vi "Test.vi"() -> ()   [LabVIEW 2018, in "Potentiostat Galvanostat.lvclass"]
uses:
  Potentiostat Galvanostat.lvclass
  Controls/OCV Parameters.ctl
  Controls/CV Parameters.ctl
  Controls/CA Parameters.ctl
  Controls/CP Parameters.ctl
  Controls/PEIS Parameters.ctl
  Controls/GEIS Parameters.ctl
  Controls/Channel Information.ctl
  Controls/Channel.ctl
  Controls/Firmware Code.ctl
  Controls/Amplifier Type.ctl
  Controls/Channel State.ctl
  Controls/Current Range.ctl
  Controls/Bandwidth.ctl
  Controls/Device Information.ctl
  Controls/Device Code.ctl
  Controls/Technique List.ctl
  Controls/PEIS-GEIS P1 Processed Data Columns.ctl
  Potentiostat Galvanostat.lvclass/Potentiostat Galvanostat.ctl
  Error Code Converter.vi
  Insert Column into Table.vi
  BL_GetErrorMsg.vi
  <vilib>/Utility/error.llb/Error Cluster From Error Code.vi
  Get Enum Size.vi
  <vilib>/Utility/Data Type/Get Numeric Information.vi
panel:
  out "Version":string="6.4.0.0"
  out "Device Information":T1={"Device Code"=36, "RAM Size"=32, "CPU"=9200, "Number Of Channels"=2, "Number Of Slots"=1, "Firmware Version"=1140, "Firmware Year"=2021, "Firmware Month"=6, "Firmware Day"=17, "HT Display On"=1, "No. of Connected PCs"=1} {"Device Code" items=["VMP device"=0, "VMP2 device"=1, "MPG device"=2, "BISTAT device"=3, "MCS-200 device"=4, "VMP3 device"=5, "VSP"=6, "HCP-803"=7, "EPP-400"=8, "EPP-4000"=9, "BISTAT 2"=10, "FCT-150S"=11, "VMP-300"=12, "SP-50"=13, "SP-150"=14, "FCT-50S"=15, "SP300"=16, "CLB-500"=17, "HCP-1005"=18, "CLB-2000"=19, "VSP-300"=20, "SP-200"=21, "MPG2"=22, "SP-100"=23, "MOSLED"=24, "Kinetic device... \\warning unused code"=25, "Nikita"=26, "SP-240"=27, "MPG-205 (techno VMP3) \\warning not controled by kernel2"=28, "MPG-210 (techno VMP3) \\warning not controled by kernel2"=29, "MPG-220 (techno VMP3) \\warning not controled by kernel2"=30, "MPG-240 (techno VMP3) \\warning not controled by kernel2"=31, "BP-300"=32, "VMP-3e  (VMP3)"=33, "VSP-3e  (VMP3)"=34, "SP-50e  (VMP3)"=35, "SP-150e (VMP3)"=36, "Unknown device"=255]}
  out "Channel Information":T3={"Channel"=0, "Board Version"=19, "Board Serial Number"=54353, "Firmware Code"=5, "Firmware Version"=5282, "Xilinx Version"=42511, "Amplifier Code"=15, "Number of Amplifiers"=0, "Low Current Board Present?"=FALSE, "Impedance Capable?"=TRUE, "RESERVED"=0, "RESERVED 2"=0, "Memory Size"=786432, "Memory Filled (in Bytes)"=0, "Channel State"=0, "Maximum Current Range Allowed"=10, "Minimum Current Range Allowed"=5, "Maximum Bandwidth"=7, "Number of Techniques"=1} {"Channel" items=["Channel 0", "Channel 1", "Channel 2", "Channel 3", "Channel 4", "Channel 5", "Channel 6", "Channel 7", "Channel 8", "Channel 9", "Channel 10", "Channel 11", "Channel 12", "Channel 13", "Channel 14", "Channel 15"]; "Firmware Code" items=["No firmware loaded"=0, "Firmware for EC-Lab software"=1, "Unknown firmware loaded"=4, "Firmware for the library"=5, "Invalid firmware loaded"=8, "Firmware for calibration software"=10]; "Amplifier Code" items=["No amplifier VMP3 series"=0, "Amplifier 2 A VMP3 series"=1, "Amplifier 1 A VMP3 series"=2, "Amplifier 5 A VMP3 series"=3, "Amplifier 10 A VMP3 series"=4, "Amplifier 20 A VMP3 series"=5, "reserved VMP3 series"=6, "Low current amplifier VMP3 series"=7, "Amplifier 80 A VMP3 series"=8, "Amplifier 4 A VMP3 series"=9, "Fuel Cell Tester VMP3 series"=10, "Amplifier 4 A (VSP instrument) VMP3 series"=11, "Low current amplifier (VSP instrument) VMP3 series"=12, "Undefined amplifier VMP3 series"=13, "reserved VMP3 series"=14, "No amplifier VMP3 series"=15, "Amplifier 8 A VMP3 series"=16, "Amplifier LB500 VMP3 series"=17, "Amplifier 100 A VMP3 series"=18, "Amplifier LB2000 VMP3 series"=19, "Amplifier 1A 48V SP-300 series"=20, "Amplifier 4A 14V SP-300 series"=21, "MPG-205 5A amplifier"=22, "MPG-210 10A amplifier"=23, "MPG-220 20A amplifier"=24, "MPG-240 40A amplifier"=25, "coin cell holder"=26, "VMP4 10A/5V amplifier (SP-300 internal amplifier)"=27, "VMP4 2A/30V"=28, "VMP4 1A/48VP"=129]; "Channel State" items=["Channel is stopped", "Channel is running", "Channel is paused"]; "Maximum Current Range Allowed" items=["I range 100 pA SP-300 series", "I range 1 nA VMP3 / SP-300 series", "I range 10 nA VMP3 / SP-300 series", "I range 100 nA VMP3 / SP-300 series", "I range 1 uA VMP3 / SP-300 series", "I range 10 uA VMP3 / SP-300 series", "I range 100 uA VMP3 / SP-300 series", "I range 1 mA VMP3 / SP-300 series", "I range 10 mA VMP3 / SP-300 series", "I range 100 mA VMP3 / SP-300 series", "I range 1 A VMP3 / SP-300 series", "Booster VMP3 / SP-300 series", "Auto range VMP3 / SP-300 series"]; "Minimum Current Range Allowed" items=["I range 100 pA SP-300 series", "I range 1 nA VMP3 / SP-300 series", "I range 10 nA VMP3 / SP-300 series", "I range 100 nA VMP3 / SP-300 series", "I range 1 uA VMP3 / SP-300 series", "I range 10 uA VMP3 / SP-300 series", "I range 100 uA VMP3 / SP-300 series", "I range 1 mA VMP3 / SP-300 series", "I range 10 mA VMP3 / SP-300 series", "I range 100 mA VMP3 / SP-300 series", "I range 1 A VMP3 / SP-300 series", "Booster VMP3 / SP-300 series", "Auto range VMP3 / SP-300 series"]; "Maximum Bandwidth" items=["Bandwidth #1"=1, "Bandwidth #2"=2, "Bandwidth #3"=3, "Bandwidth #4"=4, "Bandwidth #5"=5, "Bandwidth #6"=6, "Bandwidth #7"=7, "Bandwidth #8 (only with SP-300 series)"=8, "Bandwidth #9 (only with SP-300 series)"=9]}
  out "Plugged Channels":u8[](array[ring])=[0, 1] items=["Channel 0", "Channel 1", "Channel 2", "Channel 3", "Channel 4", "Channel 5", "Channel 6", "Channel 7", "Channel 8", "Channel 9", "Channel 10", "Channel 11", "Channel 12", "Channel 13", "Channel 14", "Channel 15"]
  in  "Stop":bool
  out "Process 1 Table":string[][](table)=[["1.000156E+5", "8.985447E-3", "1.609175E-5", "-3.228165E-1", "-8.278794E-4", "2.261308E-7", "0.000000E+0", "1.676092E-2", "1.613657E-5", "-1.723862E-1", "8.918704E-4", "-2.261308E-7", "0.000000E+0", "1.913000E+0", "1.000001E+0", "5.000068E+0", "-4.793397E+0", "-4.792189E+0", "-1.849602E+1", "-9.877000E+0", "5.583884E+2", "1.038692E+3", "2.746936E+0", "3.016487E+0", "1.771425E+2", "1.781706E+2", "5.295453E+2", "1.023296E+3"], ["7.942968E+4", "9.130012E-3", "1.555612E-5", "-3.760847E-1", "-8.272454E-4", "2.359809E-7", "0.000000E+0", "1.656449E-2", "1.558345E-5", "-2.054282E-1", "8.834808E-4", "-2.359809E-7", "0.000000E+0", "2.200000E+0", "1.000001E+0", "4.899983E+0", "-4.808099E+0", "-4.807336E+0", "-2.154807E+1", "-1.177017E+1", "5.869082E+2", "1.062954E+3", "2.768570E+0", "3.026514E+0", "2.155606E+2", "2.168281E+2", "5.458891E+2", "1.040604E+3"], ["6.309374E+4", "9.176587E-3", "1.457716E-5", "-4.301943E-1", "-8.320003E-4", "2.343205E-7", "0.000000E+0", "1.605249E-2", "1.459336E-5", "-2.420709E-1", "8.697778E-4", "-2.343205E-7", "0.000000E+0", "2.487000E+0", "1.000001E+0", "4.799986E+0", "-4.836327E+0", "-4.835845E+0", "-2.464832E+1", "-1.386964E+1", "6.295180E+2", "1.099986E+3", "2.799008E+0", "3.041387E+0", "2.625389E+2", "2.636817E+2", "5.721593E+2", "1.067915E+3"], ["5.011718E+4", "9.267574E-3", "1.345851E-5", "-4.798813E-1", "-8.280845E-4", "2.151425E-7", "0.000000E+0", "1.554337E-2", "1.346797E-5", "-2.804208E-1", "8.782047E-4", "-2.151425E-7", "0.000000E+0", "2.774000E+0", "1.000001E+0", "4.699987E+0", "-4.871003E+0", "-4.870698E+0", "-2.749517E+1", "-1.606693E+1", "6.886035E+2", "1.154099E+3", "2.837969E+0", "3.062243E+0", "3.179103E+2", "3.194085E+2", "6.108256E+2", "1.109019E+3"], ["3.981250E+4", "9.361682E-3", "1.227965E-5", "-5.128311E-1", "-8.262572E-4", "2.463346E-7", "0.000000E+0", "1.500565E-2", "1.228510E-5", "-3.115016E-1", "8.827538E-4", "-2.463346E-7", "0.000000E+0", "3.061000E+0", "1.000001E+0", "4.600019E+0", "-4.910814E+0", "-4.910621E+0", "-2.938306E+1", "-1.784773E+1", "7.623738E+2", "1.221452E+3", "2.882168E+0", "3.086876E+0", "3.740558E+2", "3.743606E+2", "6.643013E+2", "1.162668E+3"], ["3.162500E+4", "9.495218E-3", "1.114971E-5", "-5.244131E-1", "-8.288304E-4", "2.266156E-7", "0.000000E+0", "1.457268E-2", "1.115284E-5", "-3.323534E-1", "8.945179E-4", "-2.266156E-7", "0.000000E+0", "3.348000E+0", "1.000001E+0", "4.500030E+0", "-4.952736E+0", "-4.952614E+0", "-3.004666E+1", "-1.904244E+1", "8.516111E+2", "1.306634E+3", "2.930241E+0", "3.116154E+0", "4.264060E+2", "4.263136E+2", "7.371698E+2", "1.235131E+3"], ["2.511718E+4", "9.653487E-3", "1.011711E-5", "-5.154602E-1", "-8.220057E-4", "2.375851E-7", "0.000000E+0", "1.425756E-2", "1.011891E-5", "-3.393087E-1", "8.821572E-4", "-2.375851E-7", "0.000000E+0", "3.635000E+0", "1.000001E+0", "4.399971E+0", "-4.994943E+0", "-4.994866E+0", "-2.953369E+1", "-1.944096E+1", "9.541741E+2", "1.409001E+3", "2.979628E+0", "3.148911E+0", "4.703461E+2", "4.689655E+2", "8.301944E+2", "1.328667E+3"], ["1.995312E+4", "9.780001E-3", "9.222543E-6", "-4.890218E-1", "-8.317952E-4", "2.165788E-7", "0.000000E+0", "1.401417E-2", "9.223570E-6", "-3.334392E-1", "8.876571E-4", "-2.165788E-7", "0.000000E+0", "3.922000E+0", "1.000001E+0", "4.300011E+0", "-5.035149E+0", "-5.035101E+0", "-2.801888E+1", "-1.910466E+1", "1.060445E+3", "1.519386E+3", "3.025488E+0", "3.181668E+0", "4.981574E+2", "4.972872E+2", "9.361534E+2", "1.435702E+3"], ["1.585156E+4", "8.546229E-3", "7.339862E-6", "-4.445049E-1", "-8.202157E-4", "2.327903E-7", "0.000000E+0", "1.195757E-2", "7.340385E-6", "-3.115652E-1", "8.815979E-4", "-2.327904E-7", "0.000000E+0", "4.066000E+0", "1.000001E+0", "4.200072E+0", "-5.134312E+0", "-5.134281E+0", "-2.546825E+1", "-1.785137E+1", "1.164358E+3", "1.629012E+3", "3.066087E+0", "3.211924E+0", "5.006867E+2", "4.993717E+2", "1.051210E+3", "1.550583E+3"], ["1.258594E+4", "9.176141E-3", "7.330036E-6", "-3.901606E-1", "-8.220244E-4", "2.196195E-7", "0.000000E+0", "1.263255E-2", "7.330360E-6", "-2.791597E-1", "8.822691E-4", "-2.196195E-7", "0.000000E+0", "4.210000E+0", "1.000001E+0", "4.099886E+0", "-5.134894E+0", "-5.134875E+0", "-2.235455E+1", "-1.599467E+1", "1.251855E+3", "1.723320E+3", "3.097554E+0", "3.236366E+0", "4.761266E+2", "4.748572E+2", "1.157775E+3", "1.656605E+3"], ["1.001563E+4", "9.575242E-3", "7.255554E-6", "-3.389324E-1", "-8.267233E-4", "2.229029E-7", "0.000000E+0", "1.302152E-2", "7.255760E-6", "-2.448211E-1", "8.815420E-4", "-2.229029E-7", "0.000000E+0", "4.354000E+0", "1.000001E+0", "4.000678E+0", "-5.139329E+0", "-5.139317E+0", "-1.941940E+1", "-1.402721E+1", "1.319712E+3", "1.794646E+3", "3.120479E+0", "3.253979E+0", "4.387784E+2", "4.349913E+2", "1.244634E+3", "1.741131E+3"], ["7.944258E+3", "9.838177E-3", "7.131193E-6", "-2.801160E-1", "-8.239449E-4", "2.293017E-7", "0.000000E+0", "1.327432E-2", "7.131322E-6", "-2.053436E-1", "8.777387E-4", "-2.293017E-7", "0.000000E+0", "4.499000E+0", "1.000001E+0", "3.900053E+0", "-5.146838E+0", "-5.146830E+0", "-1.604946E+1", "-1.176532E+1", "1.379598E+3", "1.861411E+3", "3.139752E+0", "3.269842E+0", "3.814133E+2", "3.795483E+2", "1.325826E+3", "1.822305E+3"], ["6.310570E+3", "9.992450E-3", "7.024918E-6", "-2.357731E-1", "-8.496587E-4", "1.880729E-7", "0.000000E+0", "1.339510E-2", "7.024993E-6", "-1.738710E-1", "8.380091E-4", "-1.880729E-7", "0.000000E+0", "4.676000E+0", "1.000001E+0", "3.800069E+0", "-5.153359E+0", "-5.153354E+0", "-1.350880E+1", "-9.962077E+0", "1.422429E+3", "1.906778E+3", "3.153031E+0", "3.280300E+0", "3.322720E+2", "3.298655E+2", "1.383076E+3", "1.878028E+3"], ["5.013020E+3", "1.008475E-2", "6.978094E-6", "-1.941717E-1", "-8.439901E-4", "1.961507E-7", "0.000000E+0", "1.349288E-2", "6.978146E-6", "-1.427641E-1", "8.002557E-4", "-1.961508E-7", "0.000000E+0", "4.891000E+0", "1.000001E+0", "3.700099E+0", "-5.156263E+0", "-5.156260E+0", "-1.112522E+1", "-8.179780E+0", "1.445201E+3", "1.933591E+3", "3.159928E+0", "3.286365E+0", "2.788571E+2", "2.751105E+2", "1.418043E+3", "1.913919E+3"], ["3.981370E+3", "1.014667E-2", "6.926322E-6", "-1.626481E-1", "-8.424984E-4", "1.827560E-7", "0.000000E+0", "1.355241E-2", "6.926357E-6", "-1.222966E-1", "8.025489E-4", "-1.827560E-7", "0.000000E+0", "5.105000E+0", "1.000001E+0", "3.600032E+0", "-5.159497E+0", "-5.159495E+0", "-9.319052E+0", "-7.007077E+0", "1.464943E+3", "1.956644E+3", "3.165821E+0", "3.291512E+0", "2.372212E+2", "2.386948E+2", "1.445609E+3", "1.942030E+3"], ["3.160056E+3", "1.018775E-2", "6.921268E-6", "-1.311982E-1", "-8.471414E-4", "1.910018E-7", "0.000000E+0", "1.357444E-2", "6.921282E-6", "-9.735066E-2", "8.062589E-4", "-1.910018E-7", "0.000000E+0", "5.319000E+0", "1.000001E+0", "3.499695E+0", "-5.159814E+0", "-5.159813E+0", "-7.517101E+0", "-5.577782E+0", "1.471948E+3", "1.961262E+3", "3.167893E+0", "3.292536E+0", "1.925634E+2", "1.906287E+2", "1.459298E+3", "1.951976E+3"], ["2.514022E+3", "1.021940E-2", "6.880800E-6", "-1.155739E-1", "-8.465820E-4", "1.765624E-7", "0.000000E+0", "1.358598E-2", "6.880814E-6", "-8.642459E-2", "8.008709E-4", "-1.765624E-7", "0.000000E+0", "5.533000E+0", "1.000001E+0", "3.400369E+0", "-5.162361E+0", "-5.162360E+0", "-6.621896E+0", "-4.951764E+0", "1.485206E+3", "1.974472E+3", "3.171787E+0", "3.295451E+0", "1.712691E+2", "1.704306E+2", "1.475298E+3", "1.967103E+3"], ["1.993189E+3", "1.022407E-2", "6.874916E-6", "-1.008002E-1", "-8.456683E-4", "1.845843E-7", "0.000000E+0", "1.360339E-2", "6.874928E-6", "-7.507443E-2", "8.015048E-4", "-1.845843E-7", "0.000000E+0", "5.748000E+0", "1.000001E+0", "3.299548E+0", "-5.162733E+0", "-5.162732E+0", "-5.775424E+0", "-4.301448E+0", "1.487155E+3", "1.978695E+3", "3.172356E+0", "3.296379E+0", "1.496518E+2", "1.484099E+2", "1.479606E+3", "1.973121E+3"], ["1.582532E+3", "1.023726E-2", "6.832585E-6", "-8.925927E-2", "-8.457801E-4", "1.719544E-7", "0.000000E+0", "1.360714E-2", "6.832587E-6", "-6.638539E-2", "8.021015E-4", "-1.719544E-7", "0.000000E+0", "5.963000E+0", "1.000001E+0", "3.199352E+0", "-5.165415E+0", "-5.165415E+0", "-5.114179E+0", "-3.803603E+0", "1.498300E+3", "1.991506E+3", "3.175599E+0", "3.299182E+0", "1.335596E+2", "1.321098E+2", "1.492335E+3", "1.987119E+3"], ["1.257011E+3", "1.023577E-2", "6.865689E-6", "-8.565187E-2", "-8.428153E-4", "1.990797E-7", "0.000000E+0", "1.361169E-2", "6.865694E-6", "-6.330681E-2", "8.005354E-4", "-1.990797E-7", "0.000000E+0", "6.178000E+0", "1.000001E+0", "3.099339E+0", "-5.163316E+0", "-5.163316E+0", "-4.907491E+0", "-3.627213E+0", "1.490859E+3", "1.982566E+3", "3.173437E+0", "3.297228E+0", "1.275388E+2", "1.254261E+2", "1.485394E+3", "1.978594E+3"], ["1.001602E+3", "1.024105E-2", "6.818620E-6", "-8.622289E-2", "-8.519709E-4", "1.658540E-7", "0.000000E+0", "1.360955E-2", "6.818619E-6", "-6.351924E-2", "8.109385E-4", "-1.658541E-7", "0.000000E+0", "6.393000E+0", "1.000001E+0", "3.000695E+0", "-5.166304E+0", "-5.166304E+0", "-4.940208E+0", "-3.639384E+0", "1.501924E+3", "1.995939E+3", "3.176648E+0", "3.300147E+0", "1.293398E+2", "1.266953E+2", "1.496345E+3", "1.991914E+3"], ["7.962738E+2", "1.023797E-2", "6.800614E-6", "-8.966845E-2", "-8.586464E-4", "1.809464E-7", "0.000000E+0", "1.360620E-2", "6.800619E-6", "-6.759310E-2", "8.154316E-4", "-1.809464E-7", "0.000000E+0", "6.609000E+0", "1.000001E+0", "2.901062E+0", "-5.167452E+0", "-5.167452E+0", "-5.137624E+0", "-3.872799E+0", "1.505448E+3", "2.000730E+3", "3.177666E+0", "3.301188E+0", "1.348104E+2", "1.351326E+2", "1.499400E+3", "1.996161E+3"], ["6.310095E+2", "1.023680E-2", "6.772573E-6", "-9.970385E-2", "-8.557375E-4", "1.769541E-7", "0.000000E+0", "1.359947E-2", "6.772577E-6", "-7.368255E-2", "8.164757E-4", "-1.769541E-7", "0.000000E+0", "6.826000E+0", "1.000001E+0", "2.800036E+0", "-5.169246E+0", "-5.169246E+0", "-5.712610E+0", "-4.221699E+0", "1.511507E+3", "2.008020E+3", "3.179410E+0", "3.302768E+0", "1.504536E+2", "1.478222E+2", "1.504001E+3", "2.002571E+3"], ["5.008012E+2", "1.024276E-2", "6.778827E-6", "-1.157514E-1", "-8.594855E-4", "1.799950E-7", "0.000000E+0", "1.357695E-2", "6.778825E-6", "-8.596075E-2", "8.153943E-4", "-1.799950E-7", "0.000000E+0", "7.043000E+0", "1.000001E+0", "2.699665E+0", "-5.168845E+0", "-5.168846E+0", "-6.632066E+0", "-4.925188E+0", "1.510994E+3", "2.002847E+3", "3.179263E+0", "3.301648E+0", "1.745093E+2", "1.719542E+2", "1.500882E+3", "1.995451E+3"], ["3.985969E+2", "1.023812E-2", "6.763578E-6", "-1.358769E-1", "-8.520082E-4", "1.791368E-7", "0.000000E+0", "1.355754E-2", "6.763576E-6", "-1.017696E-1", "8.196824E-4", "-1.791368E-7", "0.000000E+0", "7.263000E+0", "1.000001E+0", "2.600534E+0", "-5.169824E+0", "-5.169824E+0", "-7.785173E+0", "-5.830967E+0", "1.513713E+3", "2.004493E+3", "3.180044E+0", "3.302005E+0", "2.050463E+2", "2.036445E+2", "1.499761E+3", "1.994122E+3"], ["3.155047E+2", "1.024478E-2", "6.695739E-6", "-1.660860E-1", "-8.559053E-4", "1.721596E-7", "0.000000E+0", "1.353332E-2", "6.695741E-6", "-1.246190E-1", "8.117215E-4", "-1.721596E-7", "0.000000E+0", "7.483000E+0", "1.000001E+0", "2.499006E+0", "-5.174201E+0", "-5.174201E+0", "-9.516024E+0", "-7.140143E+0", "1.530044E+3", "2.021183E+3", "3.184704E+0", "3.305606E+0", "2.529522E+2", "2.512263E+2", "1.508990E+3", "2.005508E+3"], ["2.516913E+2", "1.024567E-2", "6.601797E-6", "-1.972982E-1", "-8.565020E-4", "1.958895E-7", "0.000000E+0", "1.346611E-2", "6.601801E-6", "-1.477747E-1", "8.145740E-4", "-1.958896E-7", "0.000000E+0", "7.703000E+0", "1.000001E+0", "2.400868E+0", "-5.180338E+0", "-5.180338E+0", "-1.130435E+1", "-8.466866E+0", "1.551952E+3", "2.039763E+3", "3.190878E+0", "3.309580E+0", "3.042146E+2", "3.003295E+2", "1.521844E+3", "2.017532E+3"], ["1.992984E+2", "1.024235E-2", "6.482969E-6", "-2.414634E-1", "-8.555697E-4", "1.679808E-7", "0.000000E+0", "1.337553E-2", "6.482964E-6", "-1.838496E-1", "8.105283E-4", "-1.679808E-7", "0.000000E+0", "7.928000E+0", "1.000001E+0", "2.299504E+0", "-5.188226E+0", "-5.188226E+0", "-1.383484E+1", "-1.053381E+1", "1.579885E+3", "2.063182E+3", "3.198626E+0", "3.314537E+0", "3.777882E+2", "3.771820E+2", "1.534051E+3", "2.028411E+3"], ["1.586294E+2", "1.025072E-2", "6.317586E-6", "-2.838458E-1", "-8.570800E-4", "1.832597E-7", "0.000000E+0", "1.327085E-2", "6.317588E-6", "-2.150166E-1", "8.191976E-4", "-1.832597E-7", "0.000000E+0", "8.156000E+0", "1.000001E+0", "2.200384E+0", "-5.199449E+0", "-5.199449E+0", "-1.626317E+1", "-1.231954E+1", "1.622570E+3", "2.100619E+3", "3.210203E+0", "3.322347E+0", "4.544001E+2", "4.481958E+2", "1.557644E+3", "2.052248E+3"], ["1.258457E+2", "1.023991E-2", "6.074190E-6", "-3.416032E-1", "-8.607721E-4", "2.047883E-7", "0.000000E+0", "1.310643E-2", "6.074188E-6", "-2.621161E-1", "8.156926E-4", "-2.047883E-7", "0.000000E+0", "8.384000E+0", "1.000001E+0", "2.099838E+0", "-5.216512E+0", "-5.216512E+0", "-1.957242E+1", "-1.501814E+1", "1.685807E+3", "2.157726E+3", "3.226808E+0", "3.333996E+0", "5.647419E+2", "5.591205E+2", "1.588399E+3", "2.084026E+3"], ["1.001602E+2", "1.024644E-2", "5.724793E-6", "-4.031606E-1", "-8.529404E-4", "1.775697E-7", "0.000000E+0", "1.288755E-2", "5.724797E-6", "-3.132801E-1", "8.120012E-4", "-1.775697E-7", "0.000000E+0", "8.617000E+0", "1.000001E+0", "2.000695E+0", "-5.242240E+0", "-5.242240E+0", "-2.309940E+1", "-1.794963E+1", "1.789836E+3", "2.251180E+3", "3.252813E+0", "3.352410E+0", "7.022017E+2", "6.937704E+2", "1.646337E+3", "2.141610E+3"], ["7.931474E+1", "1.025435E-2", "5.329655E-6", "-4.709252E-1", "-8.507402E-4", "1.748647E-7", "0.000000E+0", "1.263690E-2", "5.329654E-6", "-3.737656E-1", "8.162519E-4", "-1.748647E-7", "0.000000E+0", "8.858000E+0", "1.000001E+0", "1.899354E+0", "-5.273301E+0", "-5.273301E+0", "-2.698203E+1", "-2.141519E+1", "1.924017E+3", "2.371056E+3", "3.284209E+0", "3.374942E+0", "8.729478E+2", "8.657284E+2", "1.714586E+3", "2.207356E+3"], ["6.316075E+1", "1.027465E-2", "4.875110E-6", "-5.177143E-1", "-8.469549E-4", "-1.204385E-7", "0.000000E+0", "1.237941E-2", "4.875107E-6", "-4.193213E-1", "8.447581E-4", "1.204385E-7", "0.000000E+0", "9.382000E+0", "1.000001E+0", "1.800447E+0", "-5.312016E+0", "-5.312016E+0", "-2.966284E+1", "-2.402534E+1", "2.107572E+3", "2.539310E+3", "3.323782E+0", "3.404716E+0", "1.043027E+3", "1.033856E+3", "1.831380E+3", "2.319318E+3"], ["5.008012E+1", "1.027394E-2", "4.353638E-6", "-5.599380E-1", "-8.529965E-4", "-1.223543E-7", "0.000000E+0", "1.208833E-2", "4.353635E-6", "-4.628955E-1", "8.469953E-4", "1.223543E-7", "0.000000E+0", "9.635000E+0", "1.000001E+0", "1.699665E+0", "-5.361148E+0", "-5.361148E+0", "-3.208208E+1", "-2.652196E+1", "2.359851E+3", "2.776606E+3", "3.372885E+0", "3.443514E+0", "1.253396E+3", "1.239868E+3", "1.999474E+3", "2.484405E+3"], ["3.985968E+1", "1.026603E-2", "3.855981E-6", "-5.749120E-1", "-8.471601E-4", "-1.167675E-7", "0.000000E+0", "1.185256E-2", "3.855982E-6", "-4.854040E-1", "8.421293E-4", "1.167674E-7", "0.000000E+0", "9.900000E+0", "1.000001E+0", "1.600534E+0", "-5.413865E+0", "-5.413865E+0", "-3.294003E+1", "-2.781160E+1", "2.662366E+3", "3.073810E+3", "3.425268E+0", "3.487677E+0", "1.447691E+3", "1.434134E+3", "2.234365E+3", "2.718744E+3"], ["3.167229E+1", "1.024885E-2", "3.403454E-6", "-5.696170E-1", "-8.559985E-4", "-1.264769E-7", "0.000000E+0", "1.164178E-2", "3.403454E-6", "-4.920622E-1", "8.488970E-4", "1.264768E-7", "0.000000E+0", "1.016700E+1", "1.000001E+0", "1.500679E+0", "-5.468080E+0", "-5.468080E+0", "-3.263665E+1", "-2.819308E+1", "3.011309E+3", "3.420576E+3", "3.478755E+0", "3.534099E+0", "1.624028E+3", "1.616032E+3", "2.535846E+3", "3.014761E+3"], ["2.516913E+1", "1.025364E-2", "3.022855E-6", "-5.465709E-1", "-8.520828E-4", "-1.275458E-7", "0.000000E+0", "1.151189E-2", "3.022856E-6", "-4.793644E-1", "8.515070E-4", "1.275457E-7", "0.000000E+0", "1.045900E+1", "1.000001E+0", "1.400868E+0", "-5.519583E+0", "-5.519583E+0", "-3.131621E+1", "-2.746556E+1", "3.392037E+3", "3.808282E+3", "3.530461E+0", "3.580729E+0", "1.763048E+3", "1.756438E+3", "2.897858E+3", "3.379044E+3"], ["1.992985E+1", "1.023266E-2", "2.718984E-6", "-4.955361E-1", "-8.502369E-4", "-1.245444E-7", "0.000000E+0", "1.140869E-2", "2.718982E-6", "-4.393786E-1", "8.477782E-4", "1.245443E-7", "0.000000E+0", "1.077400E+1", "1.000001E+0", "1.299504E+0", "-5.565593E+0", "-5.565594E+0", "-2.839213E+1", "-2.517454E+1", "3.763413E+3", "4.195942E+3", "3.575582E+0", "3.622829E+0", "1.789516E+3", "1.784858E+3", "3.310727E+3", "3.797395E+3"], ["1.583615E+1", "1.023879E-2", "2.488064E-6", "-4.378815E-1", "-8.521760E-4", "-1.239307E-7", "0.000000E+0", "1.132451E-2", "2.488065E-6", "-3.937138E-1", "8.484308E-4", "1.239306E-7", "0.000000E+0", "1.110400E+1", "1.000001E+0", "1.199649E+0", "-5.604138E+0", "-5.604138E+0", "-2.508876E+1", "-2.255814E+1", "4.115166E+3", "4.551531E+3", "3.614387E+0", "3.658158E+0", "1.744920E+3", "1.746062E+3", "3.726908E+3", "4.203297E+3"], ["1.257376E+1", "1.024008E-2", "2.336405E-6", "-3.768444E-1", "-8.305086E-4", "-1.095242E-7", "0.000000E+0", "1.129403E-2", "2.336406E-6", "-3.403211E-1", "8.468834E-4", "1.095242E-7", "0.000000E+0", "1.151600E+1", "1.000001E+0", "1.099465E+0", "-5.631452E+0", "-5.631452E+0", "-2.159159E+1", "-1.949896E+1", "4.382838E+3", "4.833931E+3", "3.641755E+0", "3.684300E+0", "1.612832E+3", "1.613517E+3", "4.075296E+3", "4.556693E+3"], ["1.001602E+1", "1.024256E-2", "2.215101E-6", "-3.188558E-1", "-8.540035E-4", "-1.246433E-7", "0.000000E+0", "1.125549E-2", "2.215102E-6", "-2.897112E-1", "8.556831E-4", "1.246432E-7", "0.000000E+0", "1.192900E+1", "1.000001E+0", "1.000695E+0", "-5.654606E+0", "-5.654606E+0", "-1.826909E+1", "-1.659923E+1", "4.623968E+3", "5.081250E+3", "3.665015E+0", "3.705971E+0", "1.449523E+3", "1.451589E+3", "4.390896E+3", "4.869496E+3"], ["7.939534E+0", "1.023145E-2", "2.142189E-6", "-2.605960E-1", "-8.313108E-4", "-1.109401E-7", "0.000000E+0", "1.123874E-2", "2.142188E-6", "-2.380843E-1", "8.559438E-4", "1.109399E-7", "0.000000E+0", "1.244600E+1", "1.000001E+0", "8.997950E-1", "-5.669142E+0", "-5.669142E+0", "-1.493105E+1", "-1.364123E+1", "4.776165E+3", "5.246384E+3", "3.679079E+0", "3.719860E+0", "1.230610E+3", "1.237315E+3", "4.614905E+3", "5.098392E+3"], ["6.300403E+0", "1.024299E-2", "2.099191E-6", "-2.098686E-1", "-8.292038E-4", "-1.121172E-7", "0.000000E+0", "1.125661E-2", "2.099190E-6", "-1.924014E-1", "8.497913E-4", "1.121170E-7", "0.000000E+0", "1.309400E+1", "1.000001E+0", "7.993683E-1", "-5.677948E+0", "-5.677948E+0", "-1.202458E+1", "-1.102379E+1", "4.879495E+3", "5.362360E+3", "3.688375E+0", "3.729356E+0", "1.016552E+3", "1.025372E+3", "4.772430E+3", "5.263413E+3"], ["5.008012E+0", "1.024216E-2", "2.059254E-6", "-1.669614E-1", "-8.240945E-4", "-1.127290E-7", "0.000000E+0", "1.124565E-2", "2.059253E-6", "-1.529838E-1", "8.446831E-4", "1.127289E-7", "0.000000E+0", "1.390600E+1", "1.000001E+0", "6.996654E-1", "-5.686290E+0", "-5.686290E+0", "-9.566185E+0", "-8.765329E+0", "4.973722E+3", "5.461035E+3", "3.696682E+0", "3.737275E+0", "8.265670E+2", "8.321951E+2", "4.904559E+3", "5.397254E+3"], ["3.977851E+0", "1.023924E-2", "2.043555E-6", "-1.407762E-1", "-8.248215E-4", "-1.144302E-7", "0.000000E+0", "1.124098E-2", "2.043554E-6", "-1.285544E-1", "8.418308E-4", "1.144301E-7", "0.000000E+0", "1.492400E+1", "1.000001E+0", "5.996485E-1", "-5.689614E+0", "-5.689614E+0", "-8.065880E+0", "-7.365625E+0", "5.010505E+3", "5.500703E+3", "3.699881E+0", "3.740418E+0", "7.030322E+2", "7.051934E+2", "4.960938E+3", "5.455312E+3"], ["3.170657E+0", "1.023057E-2", "2.035744E-6", "-1.091485E-1", "-8.409741E-4", "-1.202391E-7", "0.000000E+0", "1.123236E-2", "2.035742E-6", "-1.009806E-1", "8.629960E-4", "1.202390E-7", "0.000000E+0", "1.619800E+1", "1.000001E+0", "5.011492E-1", "-5.691277E+0", "-5.691277E+0", "-6.253749E+0", "-5.785762E+0", "5.025470E+3", "5.517575E+3", "3.701177E+0", "3.741748E+0", "5.474340E+2", "5.562215E+2", "4.995564E+3", "5.489467E+3"], ["2.504006E+0", "1.023421E-2", "2.024754E-6", "-8.639383E-2", "-8.392567E-4", "-1.154179E-7", "0.000000E+0", "1.123168E-2", "2.024752E-6", "-8.047529E-2", "8.681709E-4", "1.154178E-7", "0.000000E+0", "1.780800E+1", "1.000001E+0", "3.986354E-1", "-5.693628E+0", "-5.693628E+0", "-4.950002E+0", "-4.610895E+0", "5.054543E+3", "5.547189E+3", "3.703682E+0", "3.744073E+0", "4.361383E+2", "4.459300E+2", "5.035692E+3", "5.529236E+3"], ["1.992985E+0", "1.023889E-2", "2.021441E-6", "-6.958604E-2", "-8.443522E-4", "-1.592550E-7", "0.000000E+0", "1.123083E-2", "2.021440E-6", "-6.448835E-2", "8.737619E-4", "1.592549E-7", "0.000000E+0", "2.187000E+1", "1.000001E+0", "2.995040E-1", "-5.694339E+0", "-5.694339E+0", "-3.986986E+0", "-3.694910E+0", "5.065145E+3", "5.555857E+3", "3.704592E+0", "3.744751E+0", "3.521790E+2", "3.580398E+2", "5.052886E+3", "5.544308E+3"], ["1.584043E+0", "1.023954E-2", "2.018324E-6", "-5.549836E-2", "-8.461425E-4", "-1.598303E-7", "0.000000E+0", "1.122449E-2", "2.018323E-6", "-5.181527E-2", "8.750370E-4", "1.598302E-7", "0.000000E+0", "2.440800E+1", "1.000001E+0", "1.997669E-1", "-5.695009E+0", "-5.695009E+0", "-3.179822E+0", "-2.968796E+0", "5.073292E+3", "5.561296E+3", "3.705290E+0", "3.745176E+0", "2.814149E+2", "2.880312E+2", "5.065481E+3", "5.553832E+3"], ["1.261708E+0", "1.024052E-2", "2.016226E-6", "-4.406548E-2", "-8.456961E-4", "-1.603531E-7", "0.000000E+0", "1.122910E-2", "2.016226E-6", "-4.109204E-2", "8.743373E-4", "1.603530E-7", "0.000000E+0", "2.759200E+1", "1.000001E+0", "1.009589E-1", "-5.695461E+0", "-5.695461E+0", "-2.524766E+0", "-2.354400E+0", "5.079056E+3", "5.569368E+3", "3.705783E+0", "3.745806E+0", "2.237386E+2", "2.287923E+2", "5.074126E+3", "5.564667E+3"]]
  out "Process 0 Table":string[][](table)=[["1.000080E-1", "-3.820071E-4", "-1.028701E-7"], ["2.000160E-1", "-8.402672E-4", "-1.097473E-7"], ["3.000240E-1", "-6.875138E-4", "-1.082190E-7"], ["4.000320E-1", "-7.638904E-4", "-1.021059E-7"], ["5.000400E-1", "-5.347604E-4", "-1.043983E-7"], ["6.000480E-1", "-4.583838E-4", "-1.013418E-7"], ["7.000560E-1", "-5.347604E-4", "-1.036342E-7"], ["8.000640E-1", "-6.111371E-4", "-1.097473E-7"], ["9.000720E-1", "-4.583838E-4", "-1.005777E-7"]]
  in  "Technique Selector":T10(tab)=enum."Potentio Electrochemical Impedance Spectroscopy"
  in  "OCV Parameters":T11={"Rest duration (s)"=1.0, "Record every dE (V)"=0.01, "Record every dT (s)"=0.01, "Ewe range"=3, "CE to ground Mode"=0} {"Ewe range" items=["±2.5V", "±5V", "±10V", "Auto"]; "Record every dT (s)" min=0 format="%.2e"; "Record every dE (V)" min=0 max=100 format="%.4f"; "Rest duration (s)" min=0 format="%.2f"; "CE to ground Mode" items=["Standard", "CE to ground"]}
  in  "CV Parameters":T12={"Ei Params"={"Current step vs initial one (Ei)"=TRUE, "Voltage step (V) (Ei)"=0.0, "slew rate array (mV/s) (Ei)"=0.1}, "E1 Params"={"Current step vs initial one (E1)"=FALSE, "Voltage step (V) (E1)"=0.1, "slew rate array (mV/s) (E1)"=0.1}, "E2 Params"={"Current step vs initial one (E2)"=FALSE, "Voltage step (V) (E2)"=-0.2, "slew rate array (mV/s) (E2)"=0.1}, "Ef Params"={"Current step vs initial one (Ef)"=TRUE, "Voltage step (V) (Ef)"=0.0, "slew rate array (mV/s) (Ef)"=0.1}, "Number of cycle"=1, "recording on dE (V)"=0.01, "average every dE"=TRUE, "Begin step accumulation (1 = 100% of step)"=0.5, "End step accumulation ( 1 = 100% of step)"=0.75, "I range"=12, "Bandwidth"=5, "Ewe range"=3, "CE to ground Mode"=0} {"CE to ground Mode" items=["Standard", "CE to ground"]; "Ewe range" items=["±2.5V", "±5V", "±10V", "Auto"]; "Bandwidth" items=["1 - slow"=1, "2"=2, "3"=3, "4"=4, "5 - medium"=5, "6"=6, "7 - fast"=7]; "I range" items=["1pA", "1nA", "10nA", "100nA", "1µA", "10µA", "100µA", "1mA", "10mA", "100mA", "1A", "Booster", "Auto"]; "End step accumulation ( 1 = 100% of step)" min=0 max=1 format="%_2f"; "Begin step accumulation (1 = 100% of step)" min=0 max=1 format="%_2f"; "recording on dE (V)" min=0 max=100 format="%^_3e"; "Number of cycle" min=0 max=1000000; "Ef Params"."slew rate array (mV/s) (Ef)" min=1e-07 max=100000 format="%_5e"; "Ef Params"."Voltage step (V) (Ef)" min=-10 max=10 format="%_5e"; "E2 Params"."slew rate array (mV/s) (E2)" min=1e-07 max=100000 format="%_5e"; "E2 Params"."Voltage step (V) (E2)" min=-10 max=10 format="%_5e"; "E1 Params"."slew rate array (mV/s) (E1)" min=1e-07 max=100000 format="%_5e"; "E1 Params"."Voltage step (V) (E1)" min=-10 max=10 format="%_5e"; "Ei Params"."slew rate array (mV/s) (Ei)" min=1e-07 max=100000 format="%_5e"; "Ei Params"."Voltage step (V) (Ei)" min=-10 max=10 format="%_5e"}
  in  "CA Parameters":T13={"Voltage Steps"=[{"Voltage step vs initial one"=TRUE, "Voltage step (V)"=0.0, "Duration step (s)"=1.0}, {"Voltage step vs initial one"=TRUE, "Voltage step (V)"=0.1, "Duration step (s)"=1.0}, {"Voltage step vs initial one"=TRUE, "Voltage step (V)"=0.2, "Duration step (s)"=1.0}], "No. of steps"=2, "Record every dt (s)"=0.01, "Record every dI (A)"=1e-05, "No. of times\ntechnique is repeated"=0, "I range"=12, "Ewe range"=3, "Bandwidth"=5, "CE to ground Mode"=0} {"Voltage Steps"."Duration step (s)" min=0.001 max=80000 format="%^_3e"; "Voltage Steps"."Voltage step (V)" min=-10 max=10 format="%^_3e"; "No. of times\ntechnique is repeated" min=0 max=1000000; "No. of steps" min=0 max=99; "Record every dt (s)" min=0.0001 max=1000 format="%^_3e"; "Record every dI (A)" format="%^_3e"; "CE to ground Mode" items=["Standard", "CE to ground"]; "Ewe range" items=["±2.5V", "±5V", "±10V", "Auto"]; "Bandwidth" items=["1 - slow"=1, "2"=2, "3"=3, "4"=4, "5 - medium"=5, "6"=6, "7 - fast"=7]; "I range" items=["1pA", "1nA", "10nA", "100nA", "1µA", "10µA", "100µA", "1mA", "10mA", "100mA", "1A", "Booster", "Auto"]}
  in  "CP Parameters":T14={"Current Steps"=[{"Current step vs initial\none"=FALSE, "Current step (A)"=0.0, "Duration step (s)"=1.0}, {"Current step vs initial\none"=FALSE, "Current step (A)"=0.001, "Duration step (s)"=1.0}, {"Current step vs initial\none"=FALSE, "Current step (A)"=0.005, "Duration step (s)"=1.0}], "No. of steps"=2, "Record every dt (s)"=0.05, "Record every dE (V)"=0.005, "No. of times\ntechnique is repeated"=0, "I range"=8, "Ewe range"=3, "Bandwidth"=5, "CE to ground Mode"=0} {"Current Steps"."Duration step (s)" min=0.001 max=80000 format="%^_3e"; "Current Steps"."Current step (A)" min=-150 max=150 format="%^_3e"; "No. of times\ntechnique is repeated" min=0 max=1000000; "No. of steps" min=0 max=99; "Record every dt (s)" min=0.0001 max=1000 format="%^_3e"; "Record every dE (V)" format="%^_3e"; "CE to ground Mode" items=["Standard", "CE to ground"]; "Ewe range" items=["±2.5V", "±5V", "±10V", "Auto"]; "Bandwidth" items=["1 - slow"=1, "2"=2, "3"=3, "4"=4, "5 - medium"=5, "6"=6, "7 - fast"=7]; "I range" items=["1pA", "1nA", "10nA", "100nA", "1µA", "10µA", "100µA", "1mA", "10mA", "100mA", "1A", "Booster", "Auto"]}
  in  "PEIS Parameters":T15={"Step duration (s)"=1.0, "Record every dI (A)"=0.1, "Record every dt (s)"=0.1, "Initial voltage step (V)"=0.0, "Voltage step vs initial one"=TRUE, "Initial frequency (Hz)"=100000.0, "sweep linear/logarithmic"=FALSE, "Number of frequencies"=51, "Final frequency (Hz)"=1.0, "Sine amplitude (V)"=0.01, "No. of repeat times"=1, "No. of period to wait\nbefore each frequency"=2.0, "Non-stationary correction"=TRUE, "I Range"=12, "Bandwidth"=5, "CE to ground Mode"=0} {"CE to ground Mode" items=["Standard", "CE to ground"]; "Bandwidth" items=["1 - slow"=1, "2"=2, "3"=3, "4"=4, "5 - medium"=5, "6"=6, "7 - fast"=7]; "I Range" items=["1pA", "1nA", "10nA", "100nA", "1µA", "10µA", "100µA", "1mA", "10mA", "100mA", "1A", "Booster", "Auto"]; "No. of period to wait\nbefore each frequency" min=0 format="%.2f"; "No. of repeat times" min=1 max=1000 step=1; "Sine amplitude (V)" min=0.0005 max=0.5 format="%.2e"; "Final frequency (Hz)" min=1e-05 max=1000000 format="%.2e"; "Number of frequencies" min=1 max=10000; "Initial frequency (Hz)" min=1e-05 max=1000000 format="%.2e"; "Initial voltage step (V)" min=-10 max=10 format="%.5f"; "Record every dt (s)" min=0 format="%.2e"; "Record every dI (A)" min=0 format="%.2e"; "Step duration (s)" min=0 format="%.5f"}
  in  "GEIS Parameters":T16={"Initial frequency (Hz)"=100000.0, "sweep linear/logarithmic"=FALSE, "Number of frequencies"=51, "Final frequency (Hz)"=1.0, "Sine amplitude (A)"=0.001, "No. of repeat times"=1, "No. of period to wait\nbefore each frequency"=2.0, "Non-stationary correction"=TRUE, "I Range"=7, "Bandwidth"=5, "CE to ground Mode"=0, "Step duration (s)"=1.0, "Record every dE (V)"=0.1, "Record every dt (s)"=0.1, "Initial current step (A)"=0.0, "Current step vs initial one"=TRUE} {"Initial current step (A)" min=-10 max=10 format="%.5f"; "Record every dt (s)" min=0 format="%.2e"; "Record every dE (V)" min=0 format="%.2e"; "Step duration (s)" min=0 format="%.5f"; "CE to ground Mode" items=["Standard", "CE to ground"]; "Bandwidth" items=["1 - slow"=1, "2"=2, "3"=3, "4"=4, "5 - medium"=5, "6"=6, "7 - fast"=7]; "I Range" items=["1pA", "1nA", "10nA", "100nA", "1µA", "10µA", "100µA", "1mA", "10mA", "100mA", "1A", "Booster", "Auto"]; "No. of period to wait\nbefore each frequency" min=0 format="%.2f"; "No. of repeat times" min=1 max=1000 step=1; "Sine amplitude (A)" min=0 max=100 format="%.2e"; "Final frequency (Hz)" min=1e-05 max=1000000 format="%.2e"; "Number of frequencies" min=1 max=10000; "Initial frequency (Hz)" min=1e-05 max=1000000 format="%.2e"}
  out "Graph":cluster{"Process 1":dbl[], "Process 1":dbl[]}(graph)={"Process 1"=[529.5452530308035, 545.889084953596, 572.1593193379776, 610.8255769069101, 664.3012515496457, 737.1698372433738, 830.194371269546, 936.1533719437577, 1051.210186744779, 1157.7754464294856, 1244.6338591568729, 1325.8255112405213, 1383.076395652593, 1418.0427457237026, 1445.6089359809382, 1459.29808443306, 1475.2977294919476, 1479.6064764861203, 1492.3351868793443, 1485.3935097695417, 1496.3446575842524, 1499.3999466269931, 1504.00085953192, 1500.8824384545744, 1499.7612644501992, 1508.9901101641424, 1521.8437395105464, 1534.0511791552465, 1557.643555034983, 1588.3987117499107, 1646.3365200760659, 1714.585968940897, 1831.3804145538018, 1999.4736654113065, 2234.3645630091087, 2535.846191486877, 2897.8577039948896, 3310.7272044372244, 3726.9080724683063, 4075.295929341475, 4390.896015697206, 4614.905066128507, 4772.43040583148, 4904.558926263427, 4960.938011543006, 4995.564344908568, 5035.691614128113, 5052.886485976735, 5065.480680125493, 5074.125813710692], "Process 1"=[177.1424696636808, 215.56060545898714, 262.5388707149725, 317.91025812066243, 374.0557525179722, 426.4059831622819, 470.3460722928541, 498.1574213548436, 500.68673276134365, 476.12660501667244, 438.77841249468, 381.413324726114, 332.2720131111884, 278.85711386944, 237.22115435231407, 192.5633666913751, 171.26913286022344, 149.65176232634872, 133.559632734184, 127.53877636682385, 129.3398361198626, 134.8103782739338, 150.45355010753096, 174.50929988859426, 205.04634975076362, 252.9522145326695, 304.21460891790394, 377.7882085142731, 454.4000905559476, 564.7419242852974, 702.2017479471796, 872.94782047664, 1043.0274191423823, 1253.3962686419134, 1447.6905531373811, 1624.0278654604826, 1763.0479264760036, 1789.5156014833271, 1744.9198473348656, 1612.8322211024351, 1449.5228370584102, 1230.6099385812943, 1016.5516665522109, 826.5669840827276, 703.0321509385395, 547.4340279018801, 436.1383383136964, 352.1789799079361, 281.41486339653187, 223.73860130720374]}
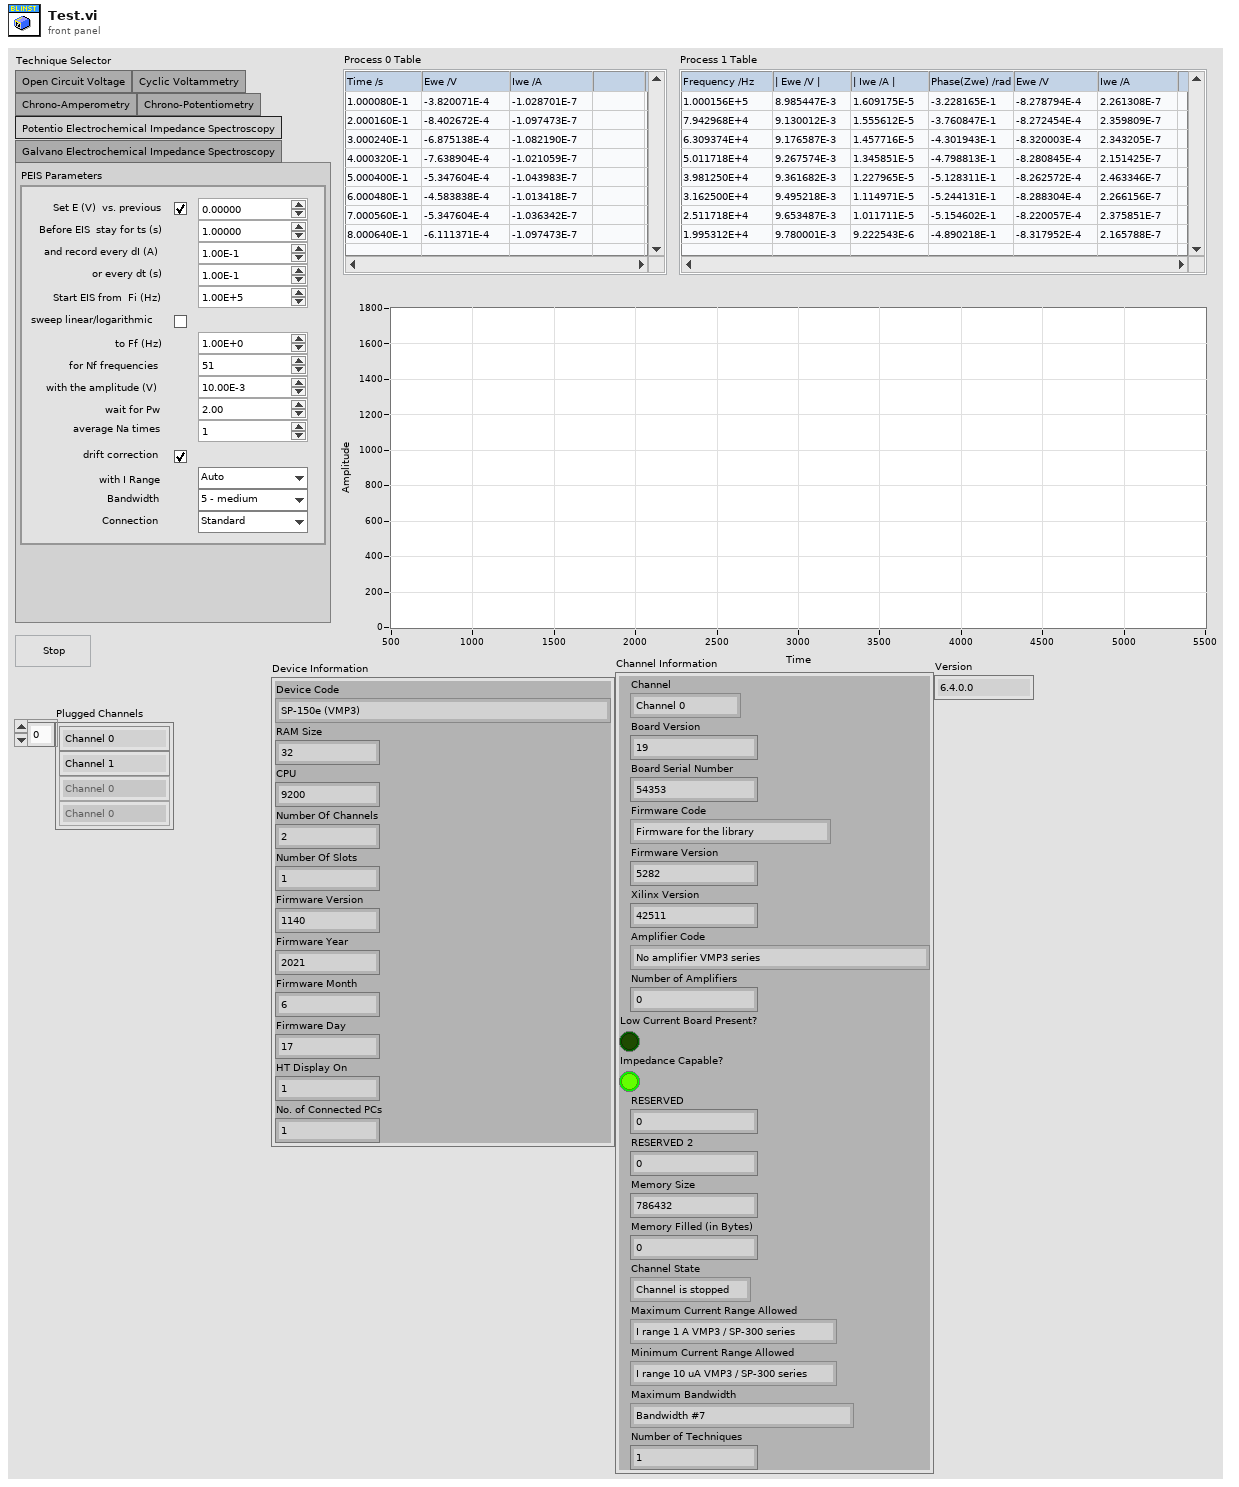
[diagram p1: front panel]
types:
  T1 = typedef "Potentiostat Galvanostat.lvclass/Device Information.ctl" = cluster{"Device Code":T2, "RAM Size":i32, "CPU":i32, "Number Of Channels":i32, "Number Of Slots":i32, "Firmware Version":i32, "Firmware Year":i32, "Firmware Month":i32, "Firmware Day":i32, "HT Display On":i32, "No. of Connected PCs":i32}
  T2 = typedef "Potentiostat Galvanostat.lvclass/Device Code.ctl" = i32
  T3 = typedef "Potentiostat Galvanostat.lvclass/Channel Information.ctl" = cluster{"Channel":T4, "Board Version":i32, "Board Serial Number":i32, "Firmware Code":T5, "Firmware Version":i32, "Xilinx Version":i32, "Amplifier Code":T6, "Number of Amplifiers":i32, "Low Current Board Present?":bool, "Impedance Capable?":bool, "RESERVED":i32, "RESERVED 2":i32, "Memory Size":i32, "Memory Filled (in Bytes)":i32, "Channel State":T7, "Maximum Current Range Allowed":T8, "Minimum Current Range Allowed":T8, "Maximum Bandwidth":T9, "Number of Techniques":i32}
  T4 = typedef "Potentiostat Galvanostat.lvclass/Channel.ctl" = u8
  T5 = typedef "Potentiostat Galvanostat.lvclass/Firmware Code.ctl" = i32
  T6 = typedef "Potentiostat Galvanostat.lvclass/Amplifier Type.ctl" = i32
  T7 = typedef "Potentiostat Galvanostat.lvclass/Channel State.ctl" = i32
  T8 = typedef "Potentiostat Galvanostat.lvclass/Current Range.ctl" = i32
  T9 = typedef "Potentiostat Galvanostat.lvclass/Bandwidth.ctl" = i32
  T10 = enum32{"Open Circuit Voltage", "Cyclic Voltammetry", "Chrono-Amperometry", "Chrono-Potentiometry", "Potentio Electrochemical Impedance Spectroscopy", "Galvano Electrochemical Impedance Spectroscopy"}
  T11 = typedef "Potentiostat Galvanostat.lvclass/OCV Parameters.ctl" = cluster{"Rest duration (s)":sgl, "Record every dE (V)":sgl, "Record every dT (s)":sgl, "Ewe range":u16, "CE to ground Mode":u16}
  T12 = typedef "Potentiostat Galvanostat.lvclass/CV Parameters.ctl" = cluster{"Ei Params":cluster{"Current step vs initial one (Ei)":bool, "Voltage step (V) (Ei)":sgl, "slew rate array (mV/s) (Ei)":sgl}, "E1 Params":cluster{"Current step vs initial one (E1)":bool, "Voltage step (V) (E1)":sgl, "slew rate array (mV/s) (E1)":sgl}, "E2 Params":cluster{"Current step vs initial one (E2)":bool, "Voltage step (V) (E2)":sgl, "slew rate array (mV/s) (E2)":sgl}, "Ef Params":cluster{"Current step vs initial one (Ef)":bool, "Voltage step (V) (Ef)":sgl, "slew rate array (mV/s) (Ef)":sgl}, "Number of cycle":i32, "recording on dE (V)":sgl, "average every dE":bool, "Begin step accumulation (1 = 100% of step)":sgl, "End step accumulation ( 1 = 100% of step)":sgl, "I range":u16, "Bandwidth":u16, "Ewe range":u16, "CE to ground Mode":u16}
  T13 = typedef "Potentiostat Galvanostat.lvclass/CA Parameters.ctl" = cluster{"Voltage Steps":cluster{"Voltage step vs initial one":bool, "Voltage step (V)":sgl, "Duration step (s)":sgl}[], "No. of steps":i32, "Record every dt (s)":sgl, "Record every dI (A)":sgl, "No. of times\ntechnique is repeated":i32, "I range":u16, "Ewe range":u16, "Bandwidth":u16, "CE to ground Mode":u16}
  T14 = typedef "Potentiostat Galvanostat.lvclass/CP Parameters.ctl" = cluster{"Current Steps":cluster{"Current step vs initial\none":bool, "Current step (A)":sgl, "Duration step (s)":sgl}[], "No. of steps":i32, "Record every dt (s)":sgl, "Record every dE (V)":sgl, "No. of times\ntechnique is repeated":i32, "I range":u16, "Ewe range":u16, "Bandwidth":u16, "CE to ground Mode":u16}
  T15 = typedef "Potentiostat Galvanostat.lvclass/PEIS Parameters.ctl" = cluster{"Step duration (s)":sgl, "Record every dI (A)":sgl, "Record every dt (s)":sgl, "Initial voltage step (V)":sgl, "Voltage step vs initial one":bool, "Initial frequency (Hz)":sgl, "sweep linear/logarithmic":bool, "Number of frequencies":i32, "Final frequency (Hz)":sgl, "Sine amplitude (V)":sgl, "No. of repeat times":i32, "No. of period to wait\nbefore each frequency":sgl, "Non-stationary correction":bool, "I Range":u16, "Bandwidth":u16, "CE to ground Mode":u16}
  T16 = typedef "Potentiostat Galvanostat.lvclass/GEIS Parameters.ctl" = cluster{"Initial frequency (Hz)":sgl, "sweep linear/logarithmic":bool, "Number of frequencies":i32, "Final frequency (Hz)":sgl, "Sine amplitude (A)":sgl, "No. of repeat times":i32, "No. of period to wait\nbefore each frequency":sgl, "Non-stationary correction":bool, "I Range":u16, "Bandwidth":u16, "CE to ground Mode":u16, "Step duration (s)":sgl, "Record every dE (V)":sgl, "Record every dt (s)":sgl, "Initial current step (A)":sgl, "Current step vs initial one":bool}
  T17 = typedef "Potentiostat Galvanostat.lvclass/Technique List.ctl" = enum16{"None", "ocv", "cv", "biovscan", "ca", "cp", "iscan", "vscan", "lasv", "load", "pow", "peis", "geis", "seisp", "seisg", "dpv", "swv", "npv", "mpv", "dnpv", "dpa", "evt", "lp", "gc", "cpp", "pdp", "psp", "zra", "ircmp", "pzir", "gzir", "loop", "TO", "TI", "TOS", "vscanlimit", "iscanlimit", "mp", "casp", "casg", "calimit", "cplimit"}
  T18 = typedef "Potentiostat Galvanostat.lvclass/PEIS-GEIS P1 Processed Data Columns.ctl" = enum16{"Frequency /Hz", "| Ewe /V |", "| Iwe /A |", "Phase(Zwe) /rad", "Ewe /V", "Iwe /A", "Ewe Range", "| Ece /V |", "| Ice /A |", "Phase(Zce) /rad", "Ece /V", "Ice /A", "Ece Range", "Time /s", "I Range", "log(| Frequuency /Hz |)", "log(| Iwe /A |)", "log(| Ice /A  |)", "Phase(Zwe) /deg", "Phase(Zce) /deg", "Zwe /ohms", "Zce /ohms", "log(| Zwe /Ohms |)", "log(| Zce /Ohms |)", "-Im(Zwe) ", "-Im(Zce)", "Re(Zwe)", "Re(Zce)"}
  T19 = typedef "Potentiostat Galvanostat.lvclass/Channel Data.ctl" = cluster{"Process Data":T20, "Data Information":T21, "Current Values":T23}
  T20 = typedef "Potentiostat Galvanostat.lvclass/Process Data.ctl" = cluster{"Process 0 Data":sgl[][], "Process 1 Data":sgl[][]}
  T21 = typedef "Potentiostat Galvanostat.lvclass/Data Information.ctl" = cluster{"Number of IRQ skipped":i32, "Buffer Row Size":i32, "Buffer Column Size":i32, "Technique Index":i32, "Technique ID":T22, "Process Index":i32, "Loop":i32, "Start Time (s)":sgl, "MuxPad":i32}
  T22 = typedef "Potentiostat Galvanostat.lvclass/Technique ID.ctl" = i32
  T23 = typedef "Potentiostat Galvanostat.lvclass/Current Values.ctl" = cluster{"State":T7, "Memory Filled (in Bytes)":i32, "Time Base (s)":sgl, "Ewe (V)":sgl, "Ewe Minimum Range (V)":sgl, "Ewe Maximum Range (V)":sgl, "Ece (V)":sgl, "Ece Minimum Range (V)":sgl, "Ece Maximum Range (V)":sgl, "E Overflow":i32, "I (A)":sgl, "I Range":T8, "I Overflow":i32, "Elapsed Time (s)":dbl, "Frequency (Hz)":sgl, "R Compensation (Ohm)":sgl, "E and/or I Saturation":sgl, "Hardware Option Error Code":T24, "Index of HW Option Error":i32}
  T24 = typedef "Potentiostat Galvanostat.lvclass/Error Codes.ctl" = i32
  T25 = typedef "Potentiostat Galvanostat.lvclass/Processed Data.ctl" = cluster{"Process 0":dbl[][], "Process 1":dbl[][]}
  T26 = typedef "Potentiostat Galvanostat.lvclass/Processed Data Column Names.ctl" = cluster{"Process 0":string[], "Process 1":string[]}
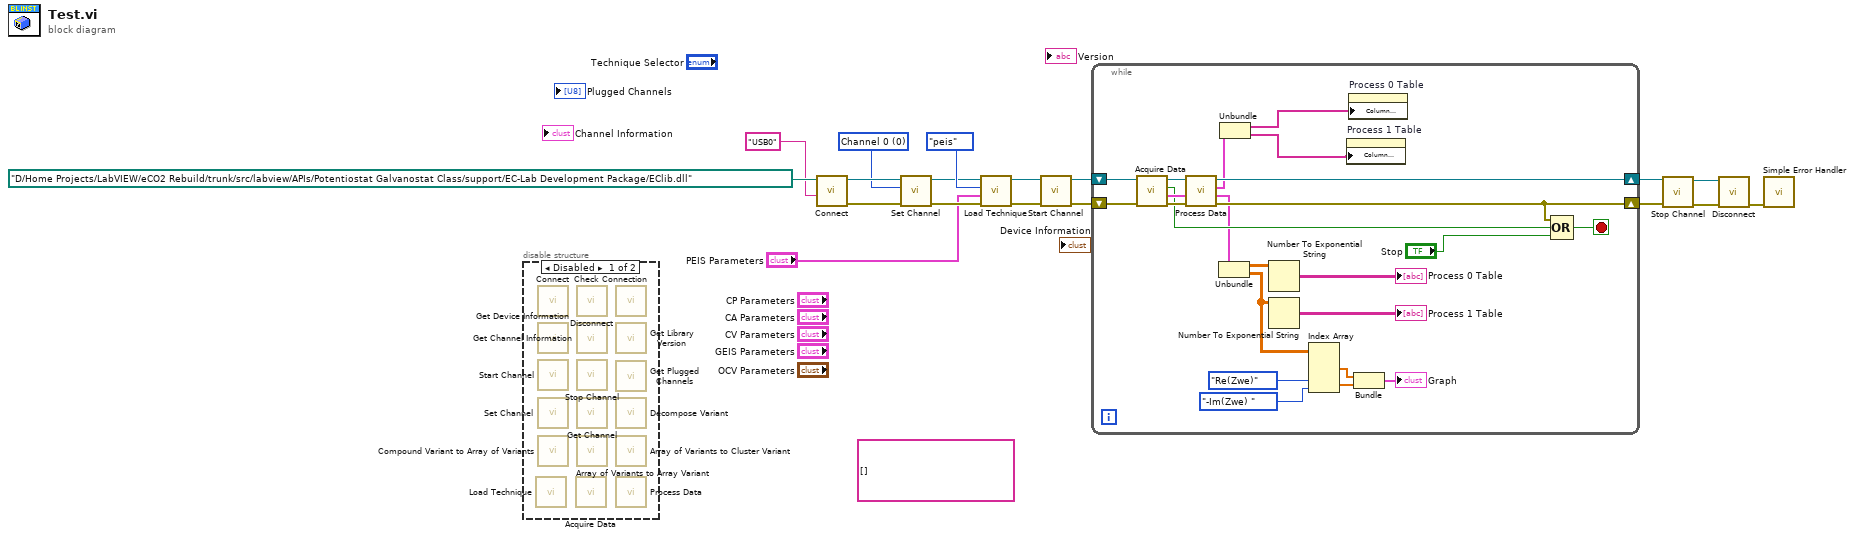
[diagram p0: block diagram]
diagram:
  (unwired) string[][] [] ("E-format string")
  w6 = T4 0 items=["Channel 0", "Channel 1", "Channel 2", "Channel 3", "Channel 4", "Channel 5", "Channel 6", "Channel 7", "Channel 8", "Channel 9", "Channel 10", "Channel 11", "Channel 12", "Channel 13", "Channel 14", "Channel 15"] ("Channel")
  n1 = disable-structure shown="Disabled" {
    frame Disabled {
      n2 = call "Load Technique.vi"() -> ()  [unwired: 10 in, 2 out]
      n3 = call "Connect.vi"() -> ()  [unwired: 10 in, 2 out]
      n4 = call "Get Device Information.vi"() -> ()  [unwired: 9 in, 3 out]
      n5 = call "Start Channel.vi"() -> ()  [unwired: 10 in, 2 out]
      n6 = call "Set Channel.vi"() -> ()  [unwired: 10 in, 2 out]
      n7 = call "Compound Variant to Array of Variants.vi"() -> ()  [unwired: 10 in, 2 out]
      n8 = call "Acquire Data.vi"() -> ()  [unwired: 8 in, 4 out]
      n9 = call "Disconnect.vi"() -> ()  [unwired: 11 in, 1 out]
      n10 = call "Get Channel Information.vi"() -> ()  [unwired: 9 in, 3 out]
      n11 = call "Stop Channel.vi"() -> ()  [unwired: 10 in, 2 out]
      n12 = call "Get Channel.vi"() -> ()  [unwired: 9 in, 3 out]
      n13 = call "Array of Variants to Array Variant.vi"() -> ()  [unwired: 10 in, 2 out]
      n14 = call "Check Connection.vi"() -> ()  [unwired: 9 in, 3 out]
      n15 = call "Get Library Version.vi"() -> ()  [unwired: 9 in, 3 out]
      n16 = call "Get Plugged Channels.vi"() -> ()  [unwired: 9 in, 3 out]
      n17 = call "Decompose Variant.vi"() -> ()  [unwired: 8 in, 4 out]
      n18 = call "Array of Variants to Cluster Variant.vi"() -> ()  [unwired: 10 in, 2 out]
      n19 = call "Process Data.vi"() -> ()  [unwired: 8 in, 4 out]
    }
    frame Enabled {
    }
  }
  n20 = call "Connect.vi"("IP Address/USB"="USB0" ("IP Address in"), ".dll Path"=path "D:/Home Projects/LabVIEW/eCO2 Rebuild/trunk/src/labview/APIs/Potentiostat Galvanostat Class/support/EC-Lab Development Package/EClib.dll" ("DLL Path in")) -> ("error out"=w8:errorcluster, "Potentiostat Galvanostat out"=w9:refnum<class "Potentiostat Galvanostat.lvclass">)  [unwired: 8 in]
  n21 = call "Set Channel.vi"("error in (no error)"=w8, "Channel"=w6, "Potentiostat Galvanostat in"=w9) -> ("error out"=w7:errorcluster, "Potentiostat Galvanostat out"=w2:refnum<class "Potentiostat Galvanostat.lvclass">)  [unwired: 7 in]
  n22 = call "Load Technique.vi"("error in (no error)"=w7, "Technique Parameters in"="PEIS Parameters", "Technique in"=Technique_List."peis", "Potentiostat Galvanostat in"=w2) -> ("error out"=w18:errorcluster, "Potentiostat Galvanostat out"=w1:refnum<class "Potentiostat Galvanostat.lvclass">)  [unwired: 6 in]
  n23 = call "Start Channel.vi"("error in (no error)"=w18, "Potentiostat Galvanostat in"=w1) -> ("error out"=w16:errorcluster, "Potentiostat Galvanostat out"=w17:refnum<class "Potentiostat Galvanostat.lvclass">)  [unwired: 8 in]
  n24 = while {
    shift-right: [w29] -> w13
    shift-left: w16 -> [w37]
    shift-right: [w38] -> w14
    shift-left: w17 -> [w41]
    stop <- w34 stop-if-true
    n25 = call "Acquire Data.vi"("error in (no error)"=w37, "Potentiostat Galvanostat in"=w41) -> ("error out"=w39:errorcluster, "Channel Data"=w31:T19, "Finished?"=w30:bool, "Potentiostat Galvanostat out"=w40:refnum<class "Potentiostat Galvanostat.lvclass">)  [unwired: 6 in]
    n26 = call "Process Data.vi"("error in (no error)"=w39, "Channel Data"=w31, "Potentiostat Galvanostat in"=w40) -> ("error out"=w29:errorcluster, "Processed Data"=w27:T25, "Column Names"=w28:T26, "Potentiostat Galvanostat out"=w38:refnum<class "Potentiostat Galvanostat.lvclass">)  [unwired: 5 in]
    n27 = Unbundle(w27) -> ("Process 0"=w26:dbl[][], "Process 1"=w25:dbl[][])
    n28 = Unbundle(w28) -> ("Process 0"=w20:string[], "Process 1"=w22:string[])
    n29 = Number To Exponential String(number=w26) -> (E-format string=→"Process 0 Table":string[][])  [unwired: 3 in]
    n30 = Number To Exponential String(number=w25) -> (E-format string=→"Process 1 Table":string[][])  [unwired: 3 in]
    n31 = Index Array(array=w25, index (col) #1=PEIS-GEIS_P1_Processed_Data_Columns."Re(Zwe)" ("PEIS"), index (col) #2=PEIS-GEIS_P1_Processed_Data_Columns."-Im(Zwe) " ("PEIS")) -> (element #1=w36:dbl[], element #2=w35:dbl[])  [unwired: 2 in]
    n32 = property on="Process 1 Table" class="Tbl (strict)"("Column Headers[]"=w22) -> ()  [unwired: 2 in, 2 out]
    n33 = property on="Process 0 Table" class="Tbl (strict)"("Column Headers[]"=w20) -> ()  [unwired: 2 in, 2 out]
    n34 = Bundle("Process 1"=w36, "Process 1"=w35) -> (→"Graph":cluster{"Process 1":dbl[], "Process 1":dbl[]})  [unwired: 1 in]
    n35 = Compound Arithmetic op=OR(w29, w30, "Stop") -> (w34:bool)
  }
  n36 = call "Stop Channel.vi"("error in (no error)"=w13, "Potentiostat Galvanostat in"=w14) -> ("error out"=w11:errorcluster, "Potentiostat Galvanostat out"=w12:refnum<class "Potentiostat Galvanostat.lvclass">)  [unwired: 8 in]
  n37 = call "Disconnect.vi"("error in (no error)"=w11, "Potentiostat Galvanostat in"=w12) -> ("error out"=w10:errorcluster)  [unwired: 9 in]
  n38 = call <vilib>:"Simple Error Handler.vi"("error in (no error)"=w10) -> ()  [unwired: 4 in, 5 out]
